vi "ReadSliderTabPosINIkeysToGFG.vi"(8 "error in (no error)":errorcluster, 11 "configuration file path":path) -> ()   [LabVIEW 2012]
doc: "SciScan 1.2 160622\nThis VI reads an INI file and stores all keys in a Generalized Functional Global Variable (GFG). It then monitors updates to the GFG and writes keys back into INI file before closing. Note that the INI file only supports data type DBL or STRING. The GFG can handle any arbitrary data type, but values that are not DBL or STRING are discarded when closing and not written to INI file."
uses:
  <vilib>/Utility/config.llb/Read Key (Double).vi
  <vilib>/Utility/config.llb/NI_LVConfig.lvlib
panel:
  out "error out":errorcluster
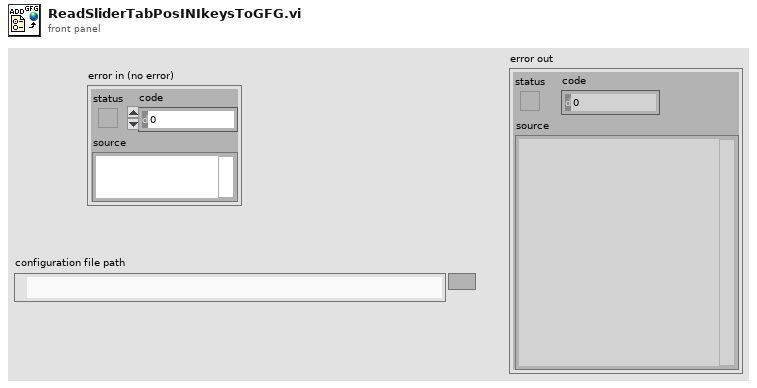
[diagram p1: front panel]
types:
  T1 = typedef "NI_LVConfig.lvlib/Config Data RefNum.ctl" = refnum<k1>
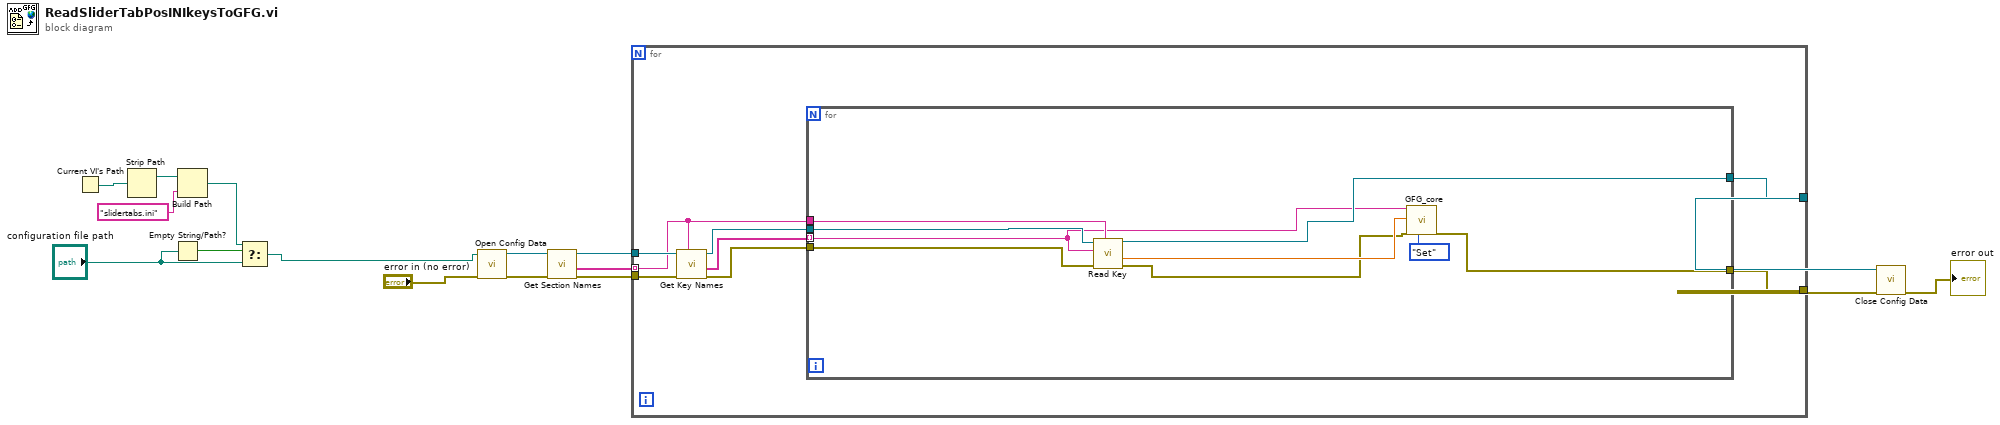
[diagram p0: block diagram]
diagram:
  n1 = Current VI's Path() -> (path=w6:path)
  n2 = Strip Path(path=w6) -> (stripped path=w7:path)  [unwired: 1 out]
  n3 = Empty String/Path?(string/path="configuration file path") -> (empty?=w5:bool)
  n4 = Build Path(base path=w7, name or relative path="slidertabs.ini") -> (appended path=w3:path)
  n5 = Select(t=w3, s=w5, f="configuration file path") -> (s? t:f=w2:path)
  n6 = call <vilib>:"Open Config Data.vi"("error in (no error)"="error in (no error)", "configuration file path"=w2) -> ("error out"=w16:errorcluster, "refnum"=w15:T1)  [unwired: 7 in, 1 out]
  n7 = call <vilib>:"Get Section Names.vi"("error in (no error)"=w16, "refnum"=w15) -> ("error out"=w14:errorcluster, "section names"=w12:string[], "refnum out"=w13:T1)  [unwired: 7 in]
  n8 = for {
    tunnel: [w23] -> w11
    tunnel: w14 -> [w21]
    tunnel: w13 -> [w20]
    tunnel: w12 -> [w18] mode=indexing
    tunnel: [w17] -> w10
    n9 = call <vilib>:"Get Key Names.vi"("section"=w18, "error in (no error)"=w21, "refnum"=w20) -> ("error out"=w22:errorcluster, "key names"=w24:string[], "refnum out"=w19:T1)  [unwired: 5 in, 1 out]
    n10 = for {
      tunnel: w19 -> [w33]
      tunnel: w18 -> [w28]
      tunnel: w24 -> [w27] mode=indexing
      tunnel: [w31] -> w23
      tunnel: w22 -> [w30]
      tunnel: [w29] -> w17
      n11 = call-poly <vilib>:"Read Key.vi"("section"=w28, "error in (no error)"=w30, "key"=w27, "refnum"=w33) -> ("error out"=w25:errorcluster, "value"=w32:dbl, "refnum out"=w31:T1)  [unwired: 4 in, 1 out]
      n12 = call "GFG_core.vi"("Variable Name in"=w27, "Variant in"=w32, "error in (no error)"=w25, "Action"=enum16{"Init", "Set", "Get"}."Set") -> ("error out"=w29:errorcluster)  [unwired: 9 in, 6 out]
    }
  }
  n13 = call <vilib>:"Close Config Data.vi"("error in (no error)"=w10, "refnum"=w11) -> ("error out"=→"error out":errorcluster)  [unwired: 8 in, 1 out]
